vi "Periodic Tasks.vi"(8 "error in":errorcluster) -> ()   [LabVIEW 2014]
doc: "This VI runs in parallel to other tasks. It can contain as many user-defined periodic loops as you need. These can carry out PID or other sorts of timed response."
uses:
  <vilib>/Platform/TimedLoop/XDataNode/timing_clust.ctl
  <vilib>/Platform/TimedLoop/XDataNode/nitl_modes.ctl
  <vilib>/Platform/TimedLoop/XDataNode/wakeup.ctl
  Global Ref.vi
  <vilib>/platform/TimedLoop/XDataNode/XDataNode.xnode
  <vilib>/Platform/TimedLoop/XDataNode/XDNodeRunTimeDep.lvlib
panel:
  in  "rate pf change Lift":dbl=5.0 format="%#_13g"
  in  "rate pf change":dbl=20.0 format="%#_13g"
  in  "Base lights hold time":dbl=5.0 format="%#_13g"
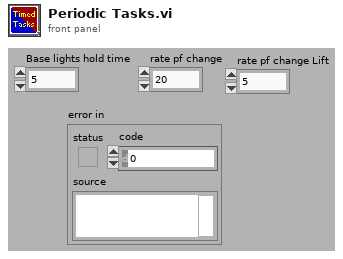
[diagram p1: front panel]
types:
  T1 = typedef "XDNodeRunTimeDep.lvlib/timing_clust.ctl" = cluster{"Expected End [f-1]":u64, "Actual End [f-1]":u64, "Finished Late? [f-1]":bool, "Expected End [i-1]":u64, "Actual End [i-1]":u64, "Finished Late? [i-1]":bool, "Expected Start [i]":u64, "Actual Start [i]":u64, "Expected Start [f]":u64, "Actual Start [f]":u64, "Source Name":string, "Structure Name":string, "Period":i64, "Deadline":i64, "Offset":i64, "Start":i64, "Priority":i32, "Timeout":i32, "Mode":T2, "Wakeup Reason":T3, "Error":errorcluster, "Source Type":string, "Secondary Source Type":string, "Global End Time":u64, "Global Start Time":u64, "Frame Duration":u64, "Iteration Duration":u64, "Assigned CPU":i32, "I/O Scan Engine Mode":u32}
  T2 = typedef "XDNodeRunTimeDep.lvlib/nitl_modes.ctl" = enum32{"No Change", "Process missed periods, maintain original phase", "Discard missed periods, maintain original phase", "Process missed periods, ignore original phase", "Discard missed periods, ignore original phase"}
  T3 = typedef "XDNodeRunTimeDep.lvlib/wakeup.ctl" = enum32{"Normal", "Aborted", "Asynchronous wakeup", "Timing source error", "Timed loop error", "Timeout"}
  T4 = typedef "WPI_JoystickDevRef.ctl" = cluster{"Device":T5}
  T5 = typedef "WPI_JoystickDeviceEnum.ctl" = enum16{"USB 0", "USB 1", "USB 2", "USB 3", "USB 4", "USB 5"}
  T6 = typedef "WPI_RobotDriveDevRef.ctl" = cluster{"DevStatus":errorcluster, "Motors[]":T7[], "Square Inputs":bool, "Max Output":dbl}
  T7 = typedef "WPI_MotorControlDeviceRef.ctl" = cluster{"DeviceStatus":errorcluster, "Type":T8, "PWM":cluster{"Controller":T9, "PWM Channel":T10, "DeadBand":T11}, "CAN":cluster{"Device Number":u8, "Control Mode":T12, "Semaphore":T13, "Max Vout":dbl, "TalonSRX Control Mode":T14}, "Invert":bool, "TransformRef":T15, "InvTransformRef":T15}
  T8 = typedef "WPI_MotorControlType.ctl" = enum16{"PWM", "CAN", "CANTalonSRX"}
  T9 = typedef "FPGA_TypedefDigitalModule.ctl" = enum16{"Controller 1"}
  T10 = typedef "FPGA_DIOPWMChannel.ctl" = enum8{"PWM 0", "PWM 1", "PWM 2", "PWM 3", "PWM 4", "PWM 5", "PWM 6", "PWM 7", "PWM 8", "PWM 9", "PWM MXP 0", "PWM MXP 1", "PWM MXP 2", "PWM MXP 3", "PWM MXP 4", "PWM MXP 5", "PWM MXP 6", "PWM MXP 7", "PWM MXP 8", "PWM MXP 9", "Invalid"}
  T11 = typedef "WPI_PWMDeadband.ctl" = cluster{"Name":string, "maxPositivePwm":i32, "minPositivePwm":i32, "centerPwm":i32, "maxNegativePwm":i32, "minNegativePwm":i32, "angularRange":u16}
  T12 = typedef "WPI_CANJaguar_ControlMode.ctl" = enum8{"Percent VBus", "Current", "Speed", "Position", "Voltage"}
  T13 = typedef "Semaphore RefNum" = refnum<k1>
  T14 = typedef "WPI_CANTalonSRX_APIControlMode.ctl" = enum8{"Percent VBus", "Speed", "Position", "Slave", "Unchanged / Invalid"}
  T15 = typedef "WPI_PWMTransform_ConPane.ctl" = refnum<vi>
  T16 = cluster{"JoystickDevRef":T4, "RobotDriveDevRef":T6}
  T17 = typedef "Global Ref typedef.ctl" = cluster{"Drive":cluster{"RobotDriveDevRef":T6}, "Joysticks":cluster{"JoyDriveRef":T4, "JoyOpRef":T4, "JoySabatourRef":T4}, "Lift":cluster{"LiftMotorRefLeft":T7, "LiftMotorRefRight":T7}, "Lift Limits":cluster{"Bottom Left":T18, "Bottom Right":T18}, "Accel":cluster{"AccelerometerDevRef":T20}, "Lift Encoder":cluster{"AIDeviceRefRight":T29, "AIDeviceRefLeft":T29}, "Lights":cluster{"Swag Light Ref cluster":cluster{"PWMDeviceRef1":T30, "PWMDeviceRef2":T30, "PWMDeviceRef3":T30, "PWMDeviceRef4":T30, "PWMDeviceRef5":T30, "PWMDeviceRef6":T30, "PWMDeviceRef7":T30, "PWMDeviceRef8":T30}}, "Camera":cluster{"GrayScaleImage":T31, "ColorImage":T31, "CameraDevRef":T32}, "Drive Encoders":cluster{"AIDeviceRef Left":T29, "AIDeviceRef Right":T29}, "Gyro":cluster{"GyroDevRef":T33}, "Relay":cluster{"RelayDevRef":T34, "RelayDevRef 2":T34}}
  T18 = typedef "WPI_DigitalInputDevRef.ctl" = cluster{"DevStatus":errorcluster, "DIO Channel":T19, "Controller":T9}
  T19 = typedef "FPGA_DIOChannel.ctl" = enum8{"DIO 0", "DIO 1", "DIO 2", "DIO 3", "DIO 4", "DIO 5", "DIO 6", "DIO 7", "DIO 8", "DIO 9", "DIO MXP 0", "DIO MXP 1", "DIO MXP 2", "DIO MXP 3", "DIO MXP 4", "DIO MXP 5", "DIO MXP 6", "DIO MXP 7", "DIO MXP 8", "DIO MXP 9", "DIO MXP 10", "DIO MXP 11", "DIO MXP 12", "DIO MXP 13", "DIO MXP 14", "DIO MXP 15", "Invalid"}
  T20 = typedef "WPI_AccelerometerDevRef.ctl" = cluster{"DevStatus":errorcluster, "Controller":T21, "Scaling":T22, "Analog Channels":T23, "I2C Bus":T25, "SPI Bus":T26, "Accel Range":T27, "ADXL345 Axes":T28, "Handle":i32, "Device Address":u8, "Accel Type":enum16{"Analog", "ADXL345 I2C", "ADXL345 SPI", "Internal"}}
  T21 = typedef "FPGA_TypedefAnalogModule.ctl" = enum16{"Controller 1"}
  T22 = typedef "WPI_AccelerometerScaling.ctl" = cluster{"Gain (VoltsPerG)":dbl, "Center Voltage":dbl}
  T23 = typedef "WPI_AccelerometerAnalogChannels.ctl" = cluster{"X-Axis":T24, "Y-Axis":T24, "Z-Axis":T24}
  T24 = typedef "FPGA_AIChannel.ctl" = enum8{"AI 0", "AI 1", "AI 2", "AI 3", "AI MXP 0", "AI MXP 1", "AI MXP 2", "AI MXP 3", "Invalid"}
  T25 = typedef "i2c_bus.ctl" = enum16{"I2C On-Board", "I2C MXP", "Invalid"}
  T26 = typedef "spi_bus.ctl" = enum16{"SPI On-Board, CS0", "SPI On-Board, CS1", "SPI On-Board, CS2", "SPI On-Board, CS3", "SPI MXP", "Invalid"}
  T27 = typedef "ADXL345 Range.ctl" = u8
  T28 = typedef "WPI_AccelerometerADXL345 Axes.ctl" = cluster{"X-Axis":bool, "Y-Axis":bool, "Z-Axis":bool}
  T29 = typedef "WPI_AnalogChannelDevRef.ctl" = cluster{"DevStatus":errorcluster, "Controller":T21, "Analog Channel":T24}
  T30 = typedef "WPI_PWMDeviceRef.ctl" = cluster{"DeviceStatus":errorcluster, "Controller":T9, "PWM Channel":T10}
  T31 = typedef "IMAQ Image.ctl" = refnum<image>
  T32 = typedef "WPI_CameraDevRef.ctl" = cluster{"Camera Address":string, "CameraStatus":errorcluster}
  T33 = typedef "WPI_GyroDevRef.ctl" = cluster{"DevStatus":errorcluster, "Analog Module":T21, "Analog Channel":T24, "Offset":dbl, "Gain (VoltsPerDegree/Second)":dbl}
  T34 = typedef "WPI_RelayDevRef.ctl" = cluster{"DevStatus":errorcluster, "Relay Channel":T35, "Controller":T9, "Relay Direction":T36}
  T35 = typedef "FPGA_DIORelayChannel.ctl" = enum8{"Relay 0", "Relay 1", "Relay 2", "Relay 3", "Invalid"}
  T36 = typedef "WPI_RelayDirection.ctl" = enum16{"Both directions", "Forward only", "Reverse only"}
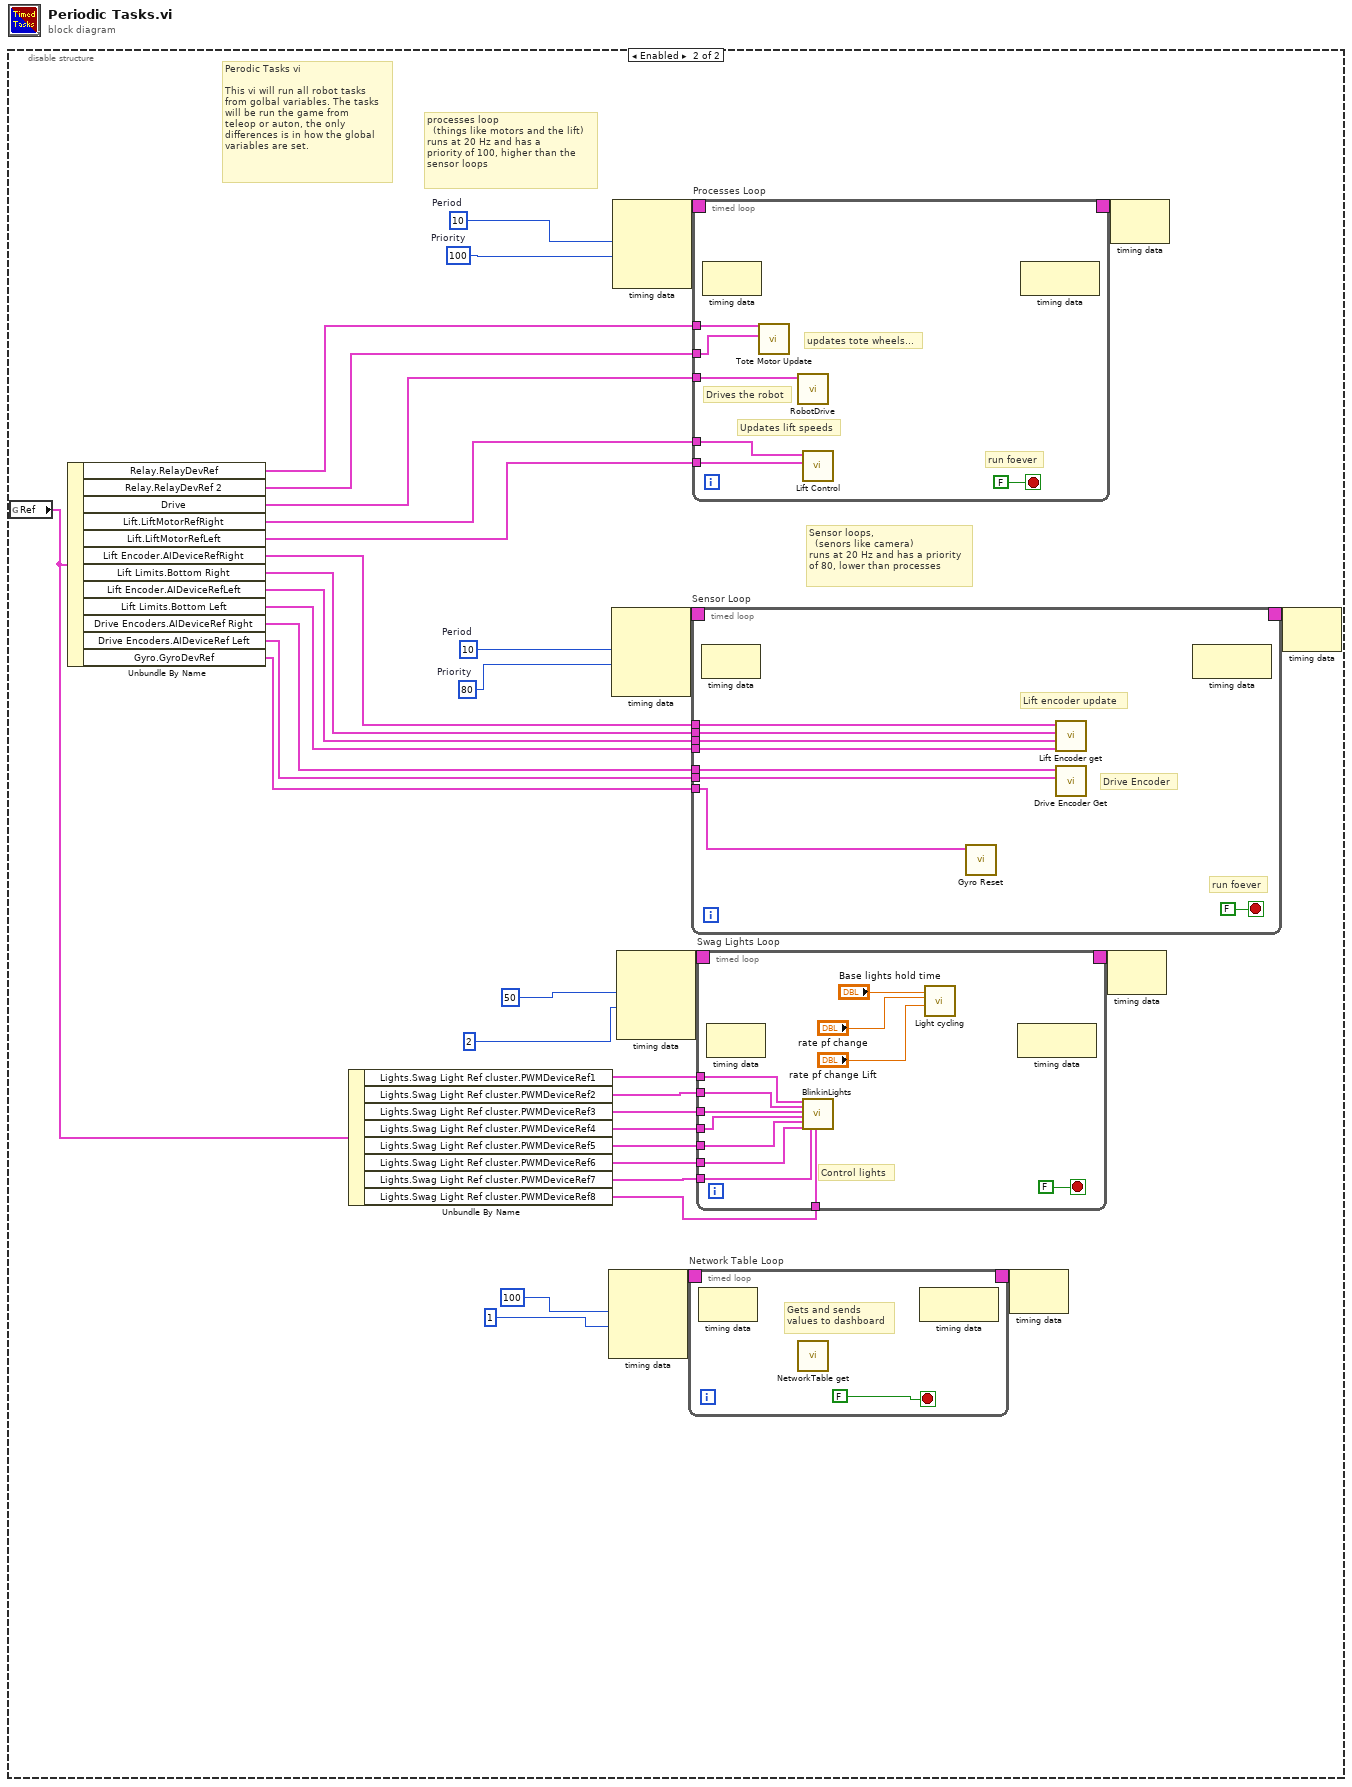
[diagram p0: block diagram]
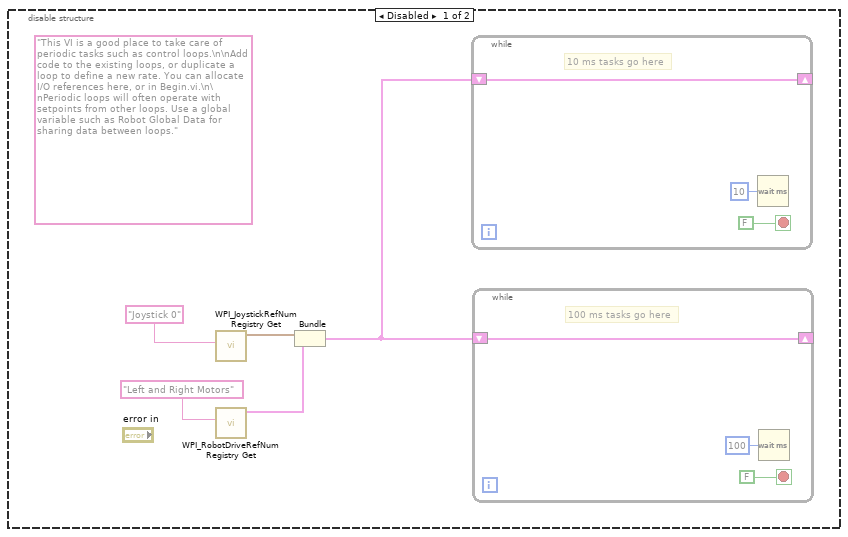
[diagram p2: hidden frame]
diagram:
  n1 = disable-structure shown="Enabled" {
    frame Disabled {
      (unwired) "This VI is a good place to take care of periodic tasks such as control loops.\n\nAdd code to the existing loops, or duplicate a loop to define a new rate. You can allocate I/O references here, or in Begin.vi.\n\nPeriodic loops will often operate with setpoints from other loops. Use a global variable such as Robot Global Data for sharing data between loops."
      n2 = call <vilib>:"WPI_JoystickRefNum Registry Get.vi"("refnum name"="Joystick 0") -> ("JoystickDevRef"=w3:T4)  [unwired: 1 in, 9 out]
      n3 = call <vilib>:"WPI_RobotDriveRefNum Registry Get.vi"("refnum name"="Left and Right Motors") -> ("RobotDriveDevRef"=w2:T6)  [unwired: 1 in, 9 out]
      n4 = Bundle("JoystickDevRef"=w3, "RobotDriveDevRef"=w2) -> (w1:T16)  [unwired: 1 out]
      n5 = while {
        shift-right: [w9] -> _
        shift-left: w1 -> [w9]
        stop <- FALSE stop-if-true
        # "10 ms tasks go here"
        n6 = Wait (ms)(milliseconds to wait=u32 10) -> ()  [unwired: 1 out]
      }
      n7 = while {
        shift-right: [w6] -> _
        shift-left: w1 -> [w6]
        stop <- FALSE stop-if-true
        # "100 ms tasks go here"
        n8 = Wait (ms)(milliseconds to wait=u32 100) -> ()  [unwired: 1 out]
      }
    }
    frame Enabled {
      w41 = 80  # Priority
      w42 = i64 10  # Period
      w45 = i64 10  # Period
      w46 = 100  # Priority
      # "Perodic Tasks vi\n\nThis vi will run all robot tasks\nfrom golbal variables. The tasks\nwill be run the game from\nteleop or auton, the only\ndifferences is in how the global\nvariables are set."
      # "Sensor loops, \n  (senors like camera)\nruns at 20 Hz and has a priority\nof 80, lower than processes"
      # "processes loop\n  (things like motors and the lift)\nruns at 20 Hz and has a\npriority of 100, higher than the\nsensor loops"
      n9 = global read "Global Ref.vi" "Ref"() -> (w17:T17)
      n10 = Unbundle By Name(w17) -> ("Relay.RelayDevRef"=w13:T34, "Relay.RelayDevRef 2"=w12:T34, "Drive"=w40:cluster{"RobotDriveDevRef":T6}, "Lift.LiftMotorRefRight"=w38:T7, "Lift.LiftMotorRefLeft"=w34:T7, "Lift Encoder.AIDeviceRefRight"=w39:T29, "Lift Limits.Bottom Right"=w37:T18, "Lift Encoder.AIDeviceRefLeft"=w33:T29, "Lift Limits.Bottom Left"=w32:T18, "Drive Encoders.AIDeviceRef Right"=w36:T29, "Drive Encoders.AIDeviceRef Left"=w35:T29, "Gyro.GyroDevRef"=w14:T33)
      n11 = Unbundle By Name(w17) -> ("Lights.Swag Light Ref cluster.PWMDeviceRef1"=w27:T30, "Lights.Swag Light Ref cluster.PWMDeviceRef2"=w26:T30, "Lights.Swag Light Ref cluster.PWMDeviceRef3"=w25:T30, "Lights.Swag Light Ref cluster.PWMDeviceRef4"=w24:T30, "Lights.Swag Light Ref cluster.PWMDeviceRef5"=w23:T30, "Lights.Swag Light Ref cluster.PWMDeviceRef6"=w22:T30, "Lights.Swag Light Ref cluster.PWMDeviceRef7"=w16:T30, "Lights.Swag Light Ref cluster.PWMDeviceRef8"=w15:T30)
      n12 = node-c288(i64 100 ("Period"), 1 ("Priority")) -> (w21:T1)  [unwired: 2 in]
      n13 = node-c288(w42, w41) -> (w44:T1)  [unwired: 2 in]
      n14 = node-c288(w45, w46) -> (w48:T1)  [unwired: 2 in]
      n15 = node-c288(i64 50 ("Period"), 2 ("Priority")) -> (w31:T1)  [unwired: 2 in]
      n16 = timed-loop "Network Table Loop" {
        timing: w21 -> [_]
        timing-out: [_] -> w20
        stop <- FALSE stop-if-true
        # "Gets and sends\nvalues to dashboard"
        n17 = node-c288() -> ()  [unwired: 1 in, 1 out]
        n18 = call "NetworkTable get.vi"() -> ()  [unwired: 12 in]
        n19 = node-c288() -> ()  [unwired: 1 in, 1 out]
      }
      n20 = timed-loop "Sensor Loop" {
        timing: w44 -> [_]
        timing-out: [_] -> w43
        tunnel: w39 -> [w82]
        tunnel: w37 -> [w81]
        tunnel: w36 -> [w80]
        tunnel: w35 -> [w79]
        tunnel: w33 -> [w78]
        tunnel: w32 -> [w77]
        tunnel: w14 -> [w76]
        stop <- FALSE stop-if-true
        # "Drive Encoder"
        # "Lift encoder update"
        # "run foever"
        n21 = node-c288() -> ()  [unwired: 1 in, 1 out]
        n22 = call "Gyro Reset.vi"("GyroDevRef"=w76) -> ()  [unwired: 11 in]
        n23 = call "Lift Encoder get.vi"("BottomSwitchRef 2"=w77, "AIDeviceRefLeft"=w78, "BottomSwitchRef"=w81, "AIDeviceRefRight"=w82) -> ()  [unwired: 8 in]
        n24 = call "Drive Encoder Get.vi"("AIDeviceRef Left"=w79, "AIDeviceRef Right"=w80) -> ()  [unwired: 10 in]
        n25 = node-c288() -> ()  [unwired: 1 in, 1 out]
      }
      n26 = timed-loop "Processes Loop" {
        timing: w48 -> [_]
        timing-out: [_] -> w47
        tunnel: w40 -> [w95]
        tunnel: w38 -> [w94]
        tunnel: w34 -> [w93]
        tunnel: w13 -> [w92]
        tunnel: w12 -> [w91]
        stop <- FALSE stop-if-true
        # "updates tote wheels..."
        # "Updates lift speeds"
        # "Drives the robot"
        # "run foever"
        n27 = node-c288() -> ()  [unwired: 1 in, 1 out]
        n28 = call "Tote Motor Update.vi"("RelayDevRef 2"=w91, "RelayDevRef"=w92) -> ()  [unwired: 10 in]
        n29 = call "RobotDrive.vi"("Drive"=w95) -> ()  [unwired: 11 in]
        n30 = call "Lift Control.vi"("MotorControlDevRefLeft"=w93, "MotorControlDevRefRight"=w94) -> ()  [unwired: 10 in]
        n31 = node-c288() -> ()  [unwired: 1 in, 1 out]
      }
      n32 = timed-loop "Swag Lights Loop" {
        timing: w31 -> [_]
        timing-out: [_] -> w30
        tunnel: w27 -> [w67]
        tunnel: w26 -> [w66]
        tunnel: w25 -> [w65]
        tunnel: w24 -> [w64]
        tunnel: w23 -> [w63]
        tunnel: w22 -> [w62]
        tunnel: w16 -> [w61]
        tunnel: w15 -> [w60]
        stop <- FALSE stop-if-true
        # "Control lights"
        n33 = node-c288() -> ()  [unwired: 1 in, 1 out]
        n34 = call "BlinkinLights.vi"("Basestrip Red"=w67, "Basestrip Green"=w66, "Basestrip Blue"=w65, "Liftstrip Red"=w64, "Liftstrip Green"=w63, "Liftstrip Blue"=w62, "Licenseplate Blue"=w61, "Licenseplate Red"=w60) -> ()  [unwired: 12 in]
        n35 = call "Light cycling.vi"("Base lights hold time"="Base lights hold time", "rate pf change Base"="rate pf change", "rate pf change Lift"="rate pf change Lift") -> ()  [unwired: 8 in]
        n36 = node-c288() -> ()  [unwired: 1 in, 1 out]
      }
      n37 = node-c288(w20) -> ()  [unwired: 1 out]
      n38 = node-c288(w30) -> ()  [unwired: 1 out]
      n39 = node-c288(w47) -> ()  [unwired: 1 out]
      n40 = node-c288(w43) -> ()  [unwired: 1 out]
    }
  }
